vi "Alert PopUUp.vi"(8 "error in (no error)":errorcluster, 11 "Pop-up Input":T1) -> (0 "error out":errorcluster)   [LabVIEW 2019, in "ZenGage v3.0 UI.lvclass"]
uses:
  ZenGage v3.0 UI.lvclass
  Common/Controls/Pop-up Input.ctl
panel:
  out "Title Display":string="Confirmation STATUS......"
  out "Message Display":string="LOGIN STATUS......"
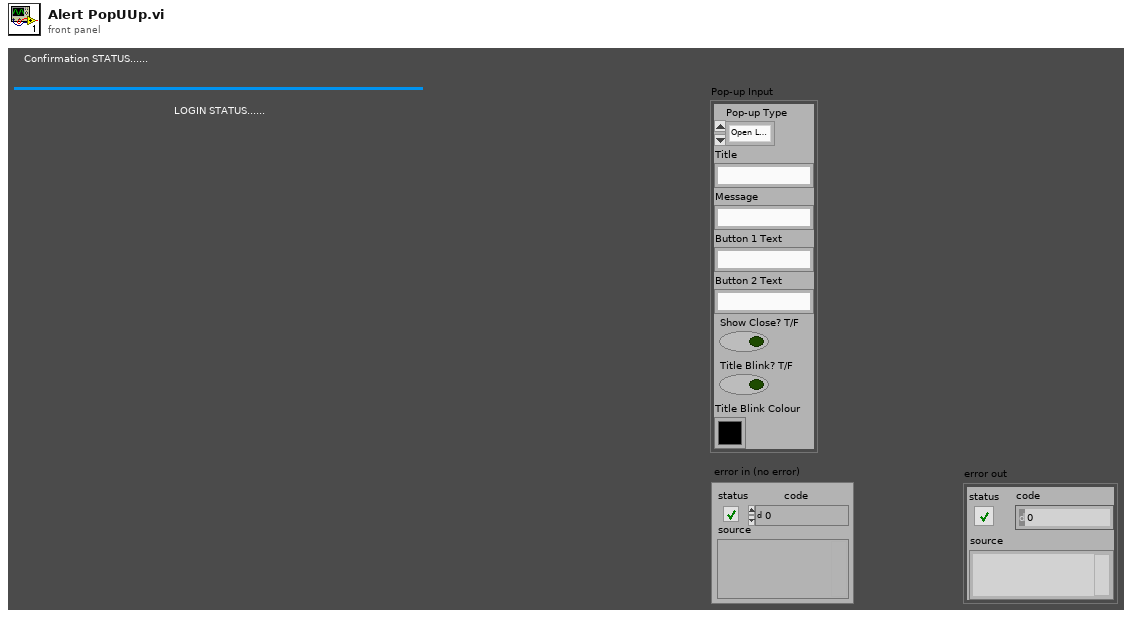
[diagram p1: front panel]
types:
  T1 = typedef "Pop-up Input.ctl" = cluster{"Pop-up Type":enum16{"Open Logo Display", "Close Logo Display", "Open Loading Bar", "Close Loading Bar", "Open Alert Display", "Close Alert Display", "One button dialog box", "Two button dialog box", "User Authentication"}, "Title":string, "Message":string, "Button 1 Text":string, "Button 2 Text":string, "Show Close? T/F":bool, "Title Blink? T/F":bool, "Title Blink Colour":u32}
  T2 = enum16{"Open Logo Display", "Close Logo Display", "Open Loading Bar", "Close Loading Bar", "Open Alert Display", "Close Alert Display", "One button dialog box", "Two button dialog box", "User Authentication"}
  T3 = enum32{"Invalid", "Standard", "Closed", "Hidden", "Minimized", "Maximized"}
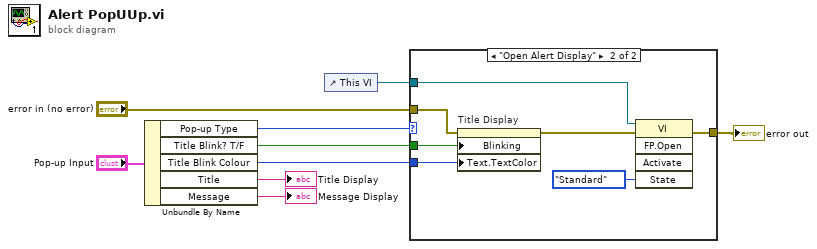
[diagram p0: block diagram]
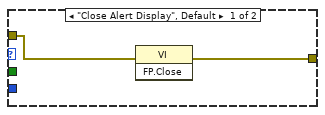
[diagram p2: hidden frame]
diagram:
  n1 = Unbundle By Name("Pop-up Input") -> ("Pop-up Type"=w1:T2, "Title Blink? T/F"=w3:bool, "Title Blink Colour"=w4:u32, "Title"=→"Title Display":string, "Message"=→"Message Display":string)
  n2 = control-ref of="This VI"() -> (w2:refnum<vi>)
  n3 = case shown="\"Open Alert Display\"" w1 {
    tunnel: "error in (no error)" -> [w11 w18]
    tunnel: [w10 w13] -> w5
    tunnel: w4 -> [_ w17]
    tunnel: w2 -> [_ w12]
    tunnel: w3 -> [_ w16]
    frame "Close Alert Display", Default {
      n4 = invoke class="VI" method="FP.Close"(error in=w11) -> (error out=w10:errorcluster)  [unwired: 2 in, 2 out]
    }
    frame "Open Alert Display" {
      n5 = property on="Title Display" class="Str"(error in=w18, "Blinking"=w16, "Text.TextColor"=w17) -> (error out=w14:errorcluster)  [unwired: 1 in, 1 out]
      n6 = invoke class="VI" method="FP.Open"(reference=w12, error in=w14, "State"=T3."Standard") -> (error out=w13:errorcluster)  [unwired: 2 in, 4 out]
    }
  }
  "error out" <- w5
